vi "LVUSBRH2_VISA_RecvResponse.vi"(8 "error in (no error)":errorcluster caption="error in(no errro)", 11 "VISA rssc":refnum<visa-resource-name>) -> (0 "error out":errorcluster, 1 "rcv string":string, 3 "VISA rssc out":refnum<visa-resource-name>)   [LabVIEW 2020]
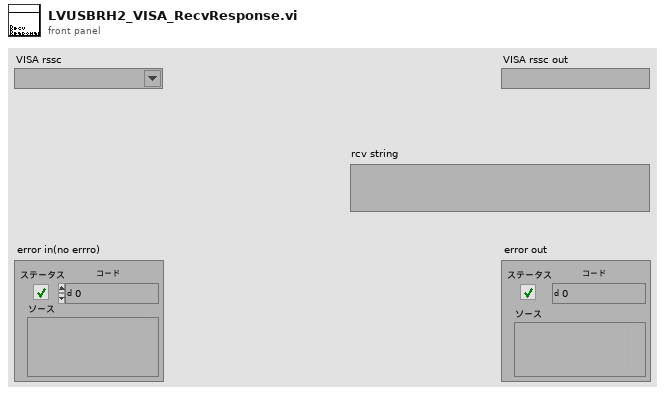
[diagram p1: front panel]
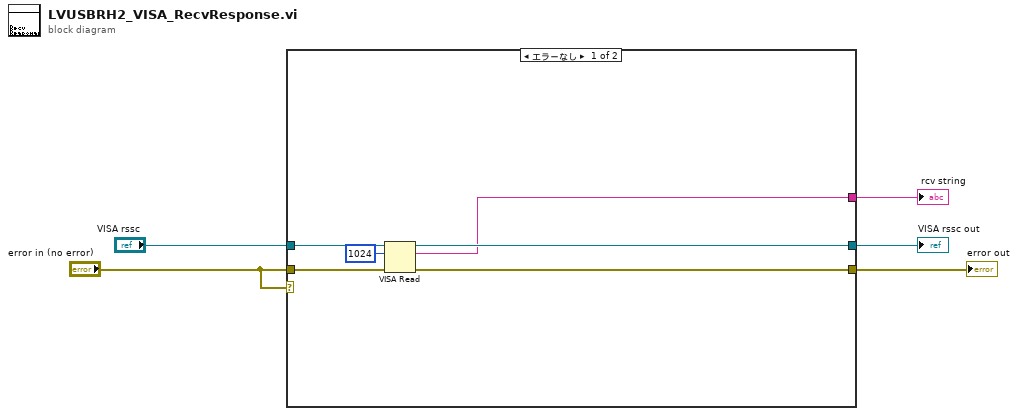
[diagram p0: block diagram]
diagram:
  n1 = case shown="エラーなし" "error in (no error)" {
    tunnel: "VISA rssc" -> [w11 w13]
    tunnel: [w10 w13] -> w4
    tunnel: "error in (no error)" -> [w9 w12]
    tunnel: [w8 w12] -> w3
    tunnel: [w7 _] -> w1
    frame No Error {
      n2 = VISA Read(VISA resource name=w11, byte count=u32 1024 ("バイトカウント"), error in (no error)=w9) -> (VISA resource name out=w10:refnum<visa-resource-name>, read buffer=w7:string, error out=w8:errorcluster)  [unwired: 1 out]
    }
    frame Error {
    }
  }
  "VISA rssc out" <- w4
  "error out" <- w3
  "rcv string" <- w1
